vi "WS1050 Delta C Calculation.vi"(8 "error in (no error)":errorcluster, 11 "Input":string[][](table)) -> (0 "error out":errorcluster, 1 "Total Bank Delta C(pF)":string[](array[string]), 2 "RTZ(pF)":string[][](array[string]), 3 "Delta C(pF)":string[][](array[string]))   [LabVIEW 2012]
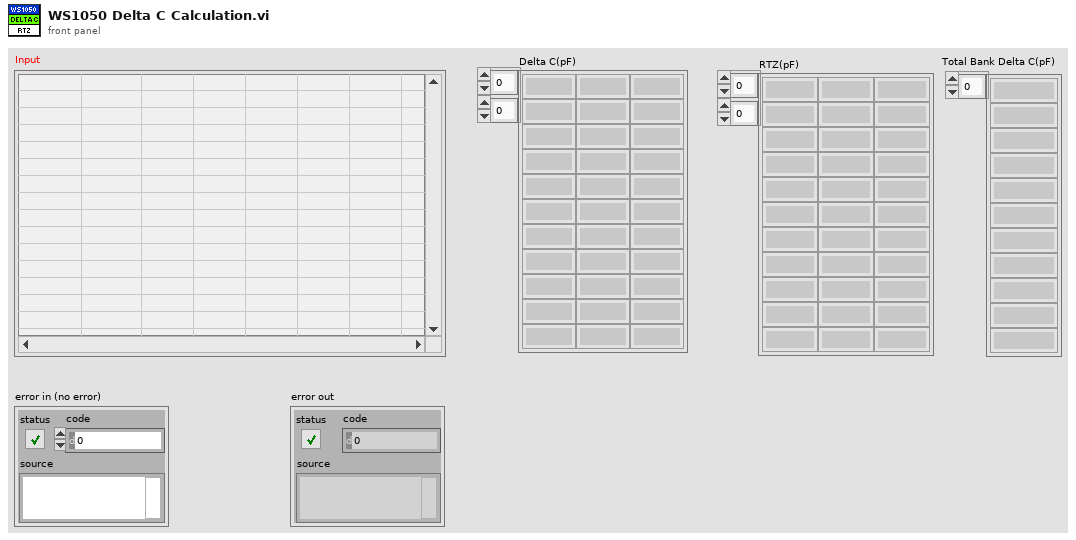
[diagram p1: front panel]
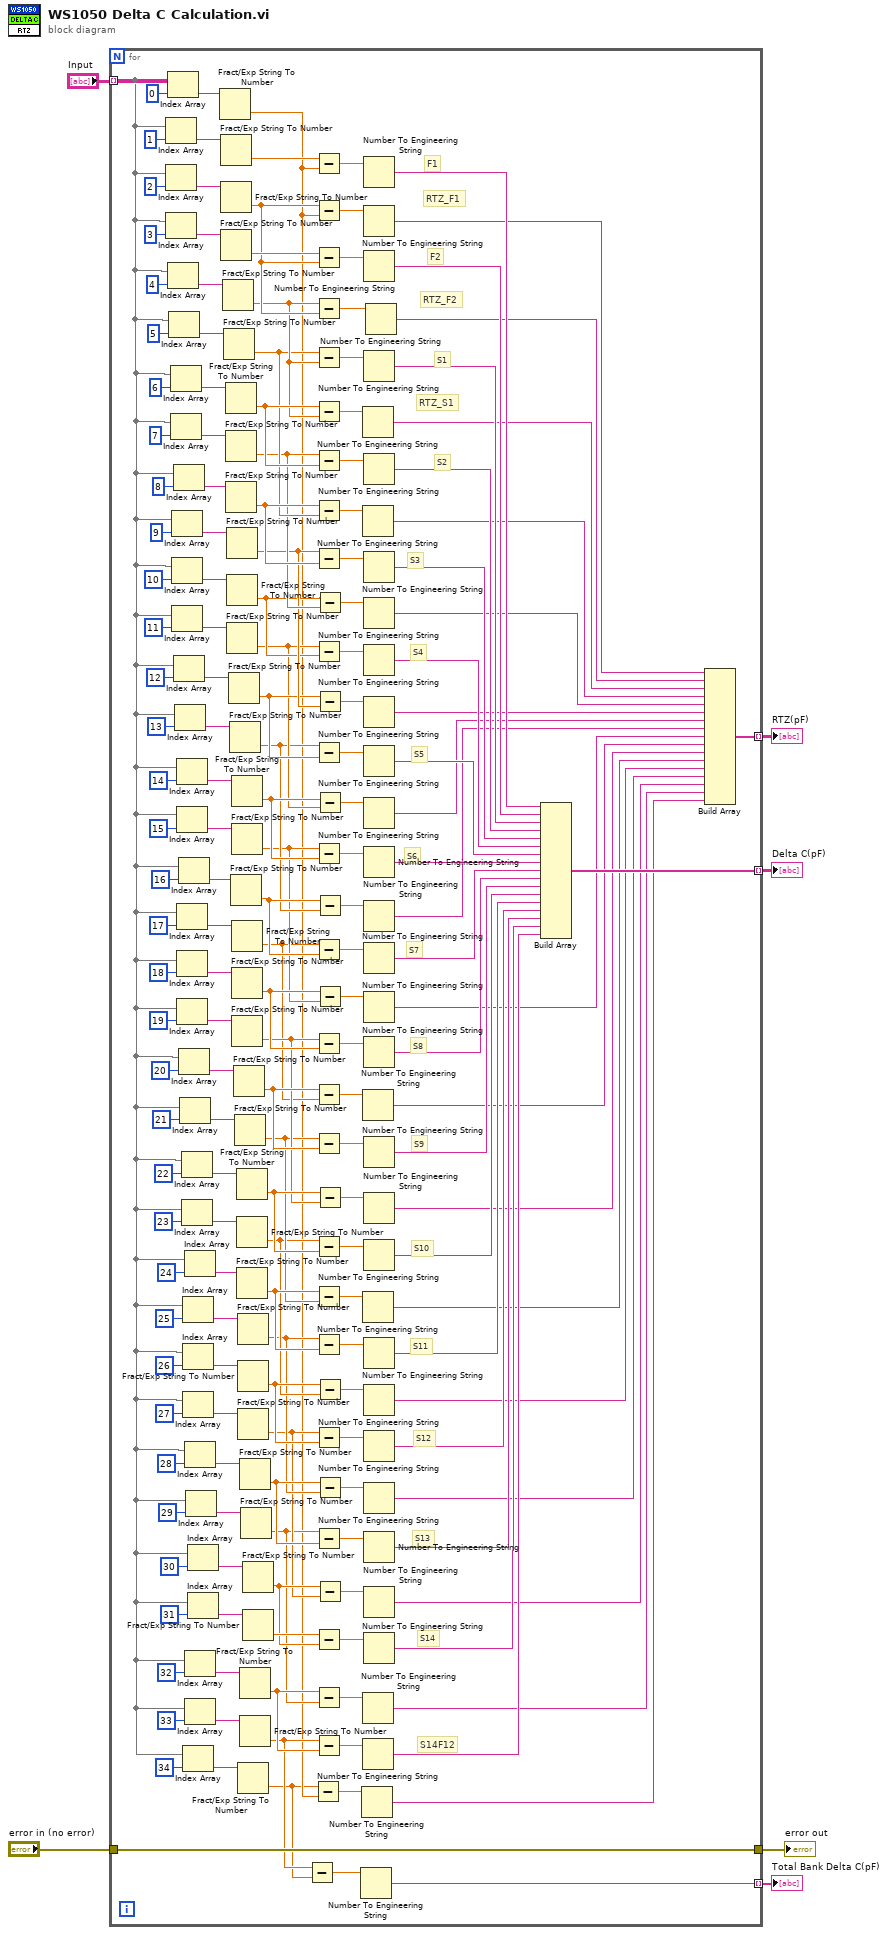
[diagram p0: block diagram]
diagram:
  n1 = for {
    tunnel: "Input" -> [w31] mode=indexing
    tunnel: [w80] -> w5 mode=indexing
    tunnel: [w13] -> w4 mode=indexing
    tunnel: "error in (no error)" -> [w12]
    tunnel: [w12] -> w2
    tunnel: [w7] -> w1 mode=indexing
    # "RTZ_S1"
    # "RTZ_F2"
    # "RTZ_F1"
    # "S14F12"
    # "S14"
    # "S13"
    # "S12"
    # "S11"
    # "S10"
    # "S9"
    # "S8"
    # "S7"
    # "S6"
    # "S5"
    # "S4"
    # "S3"
    # "S2"
    # "S1"
    # "F2"
    # "F1"
    n2 = Index Array(array=w31, index=1) -> (element=w180:string)
    n3 = Index Array(array=w31, index=2) -> (element=w179:string)
    n4 = Index Array(array=w31, index=3) -> (element=w176:string)
    n5 = Index Array(array=w31, index=0) -> (element=w181:string)
    n6 = Index Array(array=w31, index=4) -> (element=w175:string)
    n7 = Index Array(array=w31, index=5) -> (element=w172:string)
    n8 = Index Array(array=w31, index=6) -> (element=w171:string)
    n9 = Index Array(array=w31, index=7) -> (element=w168:string)
    n10 = Index Array(array=w31, index=9) -> (element=w155:string)
    n11 = Index Array(array=w31, index=10) -> (element=w156:string)
    n12 = Index Array(array=w31, index=11) -> (element=w159:string)
    n13 = Index Array(array=w31, index=8) -> (element=w154:string)
    n14 = Index Array(array=w31, index=12) -> (element=w160:string)
    n15 = Index Array(array=w31, index=13) -> (element=w163:string)
    n16 = Index Array(array=w31, index=14) -> (element=w164:string)
    n17 = Index Array(array=w31, index=15) -> (element=w167:string)
    n18 = Index Array(array=w31, index=17) -> (element=w99:string)
    n19 = Index Array(array=w31, index=18) -> (element=w100:string)
    n20 = Index Array(array=w31, index=19) -> (element=w103:string)
    n21 = Index Array(array=w31, index=16) -> (element=w98:string)
    n22 = Index Array(array=w31, index=20) -> (element=w104:string)
    n23 = Index Array(array=w31, index=21) -> (element=w107:string)
    n24 = Index Array(array=w31, index=22) -> (element=w108:string)
    n25 = Index Array(array=w31, index=23) -> (element=w111:string)
    n26 = Index Array(array=w31, index=25) -> (element=w124:string)
    n27 = Index Array(array=w31, index=26) -> (element=w123:string)
    n28 = Index Array(array=w31, index=27) -> (element=w120:string)
    n29 = Index Array(array=w31, index=34) -> (element=w32:string)
    n30 = Index Array(array=w31, index=24) -> (element=w125:string)
    n31 = Index Array(array=w31, index=28) -> (element=w119:string)
    n32 = Index Array(array=w31, index=32) -> (element=w91:string)
    n33 = Index Array(array=w31, index=33) -> (element=w94:string)
    n34 = Index Array(array=w31, index=29) -> (element=w116:string)
    n35 = Index Array(array=w31, index=30) -> (element=w115:string)
    n36 = Index Array(array=w31, index=31) -> (element=w112:string)
    n37 = Fract/Exp String To Number(string=w181) -> (number=w10:dbl)  [unwired: 3 in, 1 out]
    n38 = Fract/Exp String To Number(string=w180) -> (number=w183:dbl)  [unwired: 3 in, 1 out]
    n39 = Fract/Exp String To Number(string=w179) -> (number=w75:dbl)  [unwired: 3 in, 1 out]
    n40 = Fract/Exp String To Number(string=w176) -> (number=w150:dbl)  [unwired: 3 in, 1 out]
    n41 = Fract/Exp String To Number(string=w175) -> (number=w74:dbl)  [unwired: 3 in, 1 out]
    n42 = Fract/Exp String To Number(string=w172) -> (number=w71:dbl)  [unwired: 3 in, 1 out]
    n43 = Fract/Exp String To Number(string=w171) -> (number=w76:dbl)  [unwired: 3 in, 1 out]
    n44 = Fract/Exp String To Number(string=w168) -> (number=w69:dbl)  [unwired: 3 in, 1 out]
    n45 = Fract/Exp String To Number(string=w154) -> (number=w72:dbl)  [unwired: 3 in, 1 out]
    n46 = Fract/Exp String To Number(string=w155) -> (number=w67:dbl)  [unwired: 3 in, 1 out]
    n47 = Fract/Exp String To Number(string=w156) -> (number=w65:dbl)  [unwired: 3 in, 1 out]
    n48 = Fract/Exp String To Number(string=w159) -> (number=w53:dbl)  [unwired: 3 in, 1 out]
    n49 = Fract/Exp String To Number(string=w160) -> (number=w63:dbl)  [unwired: 3 in, 1 out]
    n50 = Fract/Exp String To Number(string=w163) -> (number=w52:dbl)  [unwired: 3 in, 1 out]
    n51 = Fract/Exp String To Number(string=w98) -> (number=w58:dbl)  [unwired: 3 in, 1 out]
    n52 = Fract/Exp String To Number(string=w164) -> (number=w61:dbl)  [unwired: 3 in, 1 out]
    n53 = Fract/Exp String To Number(string=w167) -> (number=w51:dbl)  [unwired: 3 in, 1 out]
    n54 = Fract/Exp String To Number(string=w99) -> (number=w50:dbl)  [unwired: 3 in, 1 out]
    n55 = Fract/Exp String To Number(string=w100) -> (number=w55:dbl)  [unwired: 3 in, 1 out]
    n56 = Fract/Exp String To Number(string=w103) -> (number=w54:dbl)  [unwired: 3 in, 1 out]
    n57 = Fract/Exp String To Number(string=w104) -> (number=w59:dbl)  [unwired: 3 in, 1 out]
    n58 = Fract/Exp String To Number(string=w107) -> (number=w47:dbl)  [unwired: 3 in, 1 out]
    n59 = Fract/Exp String To Number(string=w108) -> (number=w56:dbl)  [unwired: 3 in, 1 out]
    n60 = Fract/Exp String To Number(string=w111) -> (number=w44:dbl)  [unwired: 3 in, 1 out]
    n61 = Fract/Exp String To Number(string=w125) -> (number=w48:dbl)  [unwired: 3 in, 1 out]
    n62 = Fract/Exp String To Number(string=w124) -> (number=w41:dbl)  [unwired: 3 in, 1 out]
    n63 = Fract/Exp String To Number(string=w123) -> (number=w45:dbl)  [unwired: 3 in, 1 out]
    n64 = Fract/Exp String To Number(string=w120) -> (number=w38:dbl)  [unwired: 3 in, 1 out]
    n65 = Fract/Exp String To Number(string=w32) -> (number=w9:dbl)  [unwired: 3 in, 1 out]
    n66 = Fract/Exp String To Number(string=w119) -> (number=w42:dbl)  [unwired: 3 in, 1 out]
    n67 = Fract/Exp String To Number(string=w91) -> (number=w36:dbl)  [unwired: 3 in, 1 out]
    n68 = Fract/Exp String To Number(string=w94) -> (number=w11:dbl)  [unwired: 3 in, 1 out]
    n69 = Fract/Exp String To Number(string=w116) -> (number=w35:dbl)  [unwired: 3 in, 1 out]
    n70 = Fract/Exp String To Number(string=w115) -> (number=w39:dbl)  [unwired: 3 in, 1 out]
    n71 = Fract/Exp String To Number(string=w112) -> (number=w135:dbl)  [unwired: 3 in, 1 out]
    n72 = Subtract(x=w11, y=w9) -> (x-y=w8:dbl)
    n73 = Subtract(x=w9, y=w10) -> (x-y=w34:dbl)
    n74 = Subtract(x=w183, y=w10) -> (x-y=w182:dbl)
    n75 = Subtract(x=w75, y=w10) -> (x-y=w79:dbl)
    n76 = Subtract(x=w150, y=w75) -> (x-y=w151:dbl)
    n77 = Subtract(x=w74, y=w75) -> (x-y=w78:dbl)
    n78 = Subtract(x=w71, y=w74) -> (x-y=w149:dbl)
    n79 = Subtract(x=w76, y=w74) -> (x-y=w77:dbl)
    n80 = Subtract(x=w69, y=w76) -> (x-y=w148:dbl)
    n81 = Subtract(x=w72, y=w71) -> (x-y=w73:dbl)
    n82 = Subtract(x=w67, y=w72) -> (x-y=w147:dbl)
    n83 = Subtract(x=w53, y=w65) -> (x-y=w146:dbl)
    n84 = Subtract(x=w52, y=w63) -> (x-y=w145:dbl)
    n85 = Subtract(x=w51, y=w61) -> (x-y=w144:dbl)
    n86 = Subtract(x=w50, y=w58) -> (x-y=w97:dbl)
    n87 = Subtract(x=w54, y=w55) -> (x-y=w128:dbl)
    n88 = Subtract(x=w59, y=w50) -> (x-y=w60:dbl)
    n89 = Subtract(x=w47, y=w59) -> (x-y=w129:dbl)
    n90 = Subtract(x=w44, y=w56) -> (x-y=w130:dbl)
    n91 = Subtract(x=w48, y=w47) -> (x-y=w49:dbl)
    n92 = Subtract(x=w41, y=w48) -> (x-y=w131:dbl)
    n93 = Subtract(x=w38, y=w45) -> (x-y=w132:dbl)
    n94 = Subtract(x=w35, y=w42) -> (x-y=w133:dbl)
    n95 = Subtract(x=w135, y=w39) -> (x-y=w134:dbl)
    n96 = Subtract(x=w36, y=w35) -> (x-y=w37:dbl)
    n97 = Subtract(x=w11, y=w36) -> (x-y=w90:dbl)
    n98 = Subtract(x=w65, y=w69) -> (x-y=w70:dbl)
    n99 = Subtract(x=w63, y=w67) -> (x-y=w68:dbl)
    n100 = Subtract(x=w61, y=w53) -> (x-y=w66:dbl)
    n101 = Subtract(x=w58, y=w52) -> (x-y=w64:dbl)
    n102 = Subtract(x=w55, y=w51) -> (x-y=w62:dbl)
    n103 = Subtract(x=w56, y=w54) -> (x-y=w57:dbl)
    n104 = Subtract(x=w45, y=w44) -> (x-y=w46:dbl)
    n105 = Subtract(x=w42, y=w41) -> (x-y=w43:dbl)
    n106 = Subtract(x=w39, y=w38) -> (x-y=w40:dbl)
    n107 = Number To Engineering String(4:w8) -> (0:w7:string)  [unwired: 3 in]
    n108 = Number To Engineering String(4:w34) -> (0:w14:string)  [unwired: 3 in]
    n109 = Number To Engineering String(4:w77) -> (0:w28:string)  [unwired: 3 in]
    n110 = Number To Engineering String(4:w73) -> (0:w27:string)  [unwired: 3 in]
    n111 = Number To Engineering String(4:w60) -> (0:w21:string)  [unwired: 3 in]
    n112 = Number To Engineering String(4:w49) -> (0:w19:string)  [unwired: 3 in]
    n113 = Number To Engineering String(4:w37) -> (0:w15:string)  [unwired: 3 in]
    n114 = Number To Engineering String(4:w90) -> (0:w81:string)  [unwired: 3 in]
    n115 = Number To Engineering String(4:w182) -> (0:w143:string)  [unwired: 3 in]
    n116 = Number To Engineering String(4:w79) -> (0:w30:string)  [unwired: 3 in]
    n117 = Number To Engineering String(4:w151) -> (0:w142:string)  [unwired: 3 in]
    n118 = Number To Engineering String(4:w149) -> (0:w141:string)  [unwired: 3 in]
    n119 = Number To Engineering String(4:w148) -> (0:w140:string)  [unwired: 3 in]
    n120 = Number To Engineering String(4:w147) -> (0:w139:string)  [unwired: 3 in]
    n121 = Number To Engineering String(4:w70) -> (0:w26:string)  [unwired: 3 in]
    n122 = Number To Engineering String(4:w146) -> (0:w138:string)  [unwired: 3 in]
    n123 = Number To Engineering String(4:w68) -> (0:w25:string)  [unwired: 3 in]
    n124 = Number To Engineering String(4:w145) -> (0:w137:string)  [unwired: 3 in]
    n125 = Number To Engineering String(4:w66) -> (0:w24:string)  [unwired: 3 in]
    n126 = Number To Engineering String(4:w144) -> (0:w136:string)  [unwired: 3 in]
    n127 = Number To Engineering String(4:w64) -> (0:w23:string)  [unwired: 3 in]
    n128 = Number To Engineering String(4:w97) -> (0:w89:string)  [unwired: 3 in]
    n129 = Number To Engineering String(4:w62) -> (0:w22:string)  [unwired: 3 in]
    n130 = Number To Engineering String(4:w128) -> (0:w88:string)  [unwired: 3 in]
    n131 = Number To Engineering String(4:w129) -> (0:w87:string)  [unwired: 3 in]
    n132 = Number To Engineering String(4:w57) -> (0:w20:string)  [unwired: 3 in]
    n133 = Number To Engineering String(4:w130) -> (0:w86:string)  [unwired: 3 in]
    n134 = Number To Engineering String(4:w131) -> (0:w85:string)  [unwired: 3 in]
    n135 = Number To Engineering String(4:w46) -> (0:w18:string)  [unwired: 3 in]
    n136 = Number To Engineering String(4:w132) -> (0:w84:string)  [unwired: 3 in]
    n137 = Number To Engineering String(4:w43) -> (0:w17:string)  [unwired: 3 in]
    n138 = Number To Engineering String(4:w133) -> (0:w83:string)  [unwired: 3 in]
    n139 = Number To Engineering String(4:w40) -> (0:w16:string)  [unwired: 3 in]
    n140 = Number To Engineering String(4:w134) -> (0:w82:string)  [unwired: 3 in]
    n141 = Number To Engineering String(4:w78) -> (0:w29:string)  [unwired: 3 in]
    n142 = Build Array(w143, w142, w141, w140, w139, w138, w137, w136, w89, w88, w87, w86, w85, w84, w83, w82, w81) -> (w80:string[])
    n143 = Build Array(w30, w29, w28, w27, w26, w25, w24, w23, w22, w21, w20, w19, w18, w17, w16, w15, w14) -> (w13:string[])
  }
  "Delta C(pF)" <- w5
  "RTZ(pF)" <- w4
  "error out" <- w2
  "Total Bank Delta C(pF)" <- w1
